vi "aerial phase.vi"(3 "aerial condition":T1={"pini"=0.0, "vi"=0.0, "pf"=0.0, "vf"=0.0, "t"=0.0, "a"=0.1}) -> (0 "time180":dbl, 1 "flight_C":dbl[](array[numeric]))   [LabVIEW 2019]
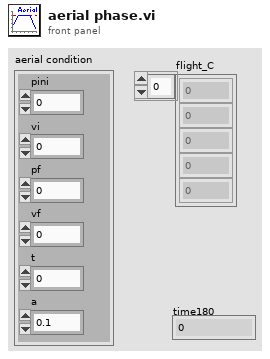
[diagram p1: front panel]
types:
  T1 = cluster{"pini":dbl, "vi":dbl, "pf":dbl, "vf":dbl, "t":dbl, "a":dbl}
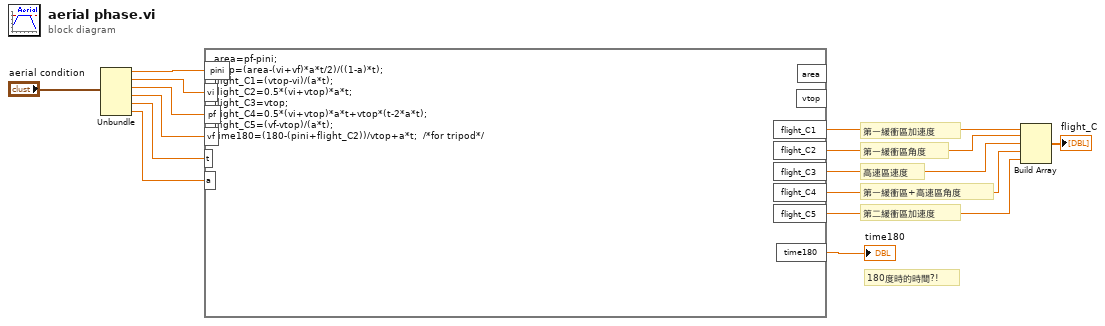
[diagram p0: block diagram]
diagram:
  # "180度時的時間?!"
  # "第二緩衝區加速度"
  # "第一緩衝區+高速區角度"
  # "高速區速度"
  # "第一緩衝區角度"
  # "第一緩衝區加速度"
  n1 = Unbundle("aerial condition") -> ("pini"=w13:dbl, "vi"=w12:dbl, "pf"=w11:dbl, "vf"=w10:dbl, "t"=w9:dbl, "a"=w8:dbl)
  n2 = formula code="area=pf-pini;\nvtop=(area-(vi+vf)*a*t/2)/((1-a)*t);\nflight_C1=(vtop-vi)/(a*t);\nflight_C2=0.5*(vi+vtop)*a*t; \nflight_C3=vtop;\nflight_C4=0.5*(vi+vtop)*a*t+vtop*(t-2*a*t);\nflight_C5=(vf-vtop)/(a*t);\ntime180=(180-(pini+flight_C2))/vtop+a*t;  /*for tripod*/"("pini"=w13, "vi"=w12, "pf"=w11, "vf"=w10, "t"=w9, "a"=w8) -> ("flight_C1"=w7:dbl, "flight_C2"=w6:dbl, "flight_C3"=w5:dbl, "flight_C4"=w4:dbl, "flight_C5"=w3:dbl, "time180"=→"time180":dbl)  [unwired: 2 out]
  n3 = Build Array(w7, w6, w5, w4, w3) -> (→"flight_C":dbl[])
